vi "addObserver.vi"(8 "error in (no error)":errorcluster, 10 "Observer.lvclass":refnum<class "Observer.lvclass">, 11 "Observable in":refnum<class "Observable.lvclass">) -> (0 "error out":errorcluster, 3 "Observable out":refnum<class "Observable.lvclass">)   [LabVIEW 2020, in "Observable.lvclass"]
uses:
  Observable.lvclass
  Observer/Observer.lvclass
  Observable.lvclass/Observable.ctl
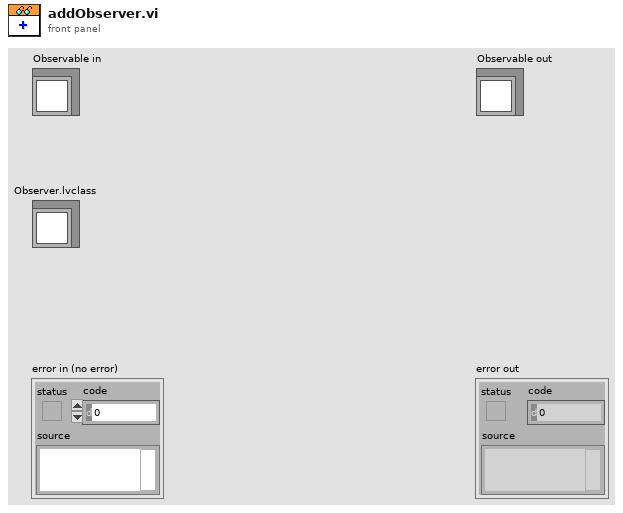
[diagram p1: front panel]
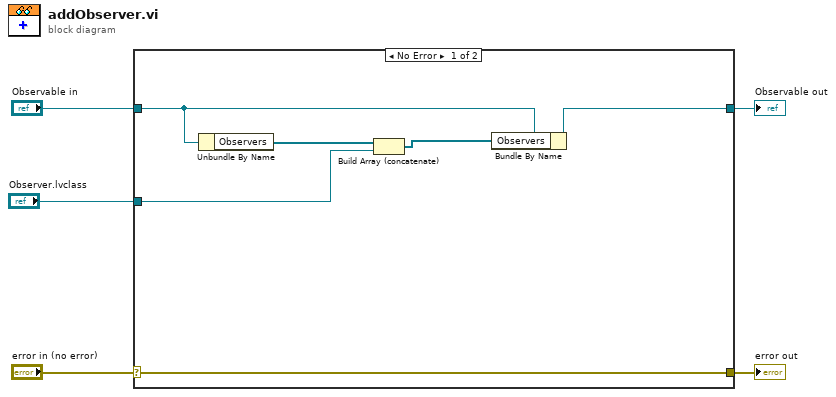
[diagram p0: block diagram]
diagram:
  n1 = case shown="No Error" "error in (no error)" {
    selector: "error in (no error)" -> [w11 w13]
    tunnel: [w11 w13] -> w4
    tunnel: [w8 w12] -> w2
    tunnel: "Observable in" -> [w10 w12]
    tunnel: "Observer.lvclass" -> [w7 _]
    frame No Error {
      n2 = Unbundle By Name(w10) -> ("Observers"=w9:refnum<class "Observer.lvclass">[])
      n3 = Build Array (concatenate)(w9, w7) -> (w6:refnum<class "Observer.lvclass">[])
      n4 = Bundle By Name(cluster=w10, "Observers"=w6) -> (w8:refnum<class "Observable.lvclass">)
    }
    frame Error {
    }
  }
  "error out" <- w4
  "Observable out" <- w2
